vi "GenerateUUID.vi"(8 "error in (no error)":errorcluster) -> (0 "error out":errorcluster, 2 "UUID":string)   [LabVIEW 2019, in "Memory Data Access.lvlib"]
uses:
  Memory Data Access.lvlib
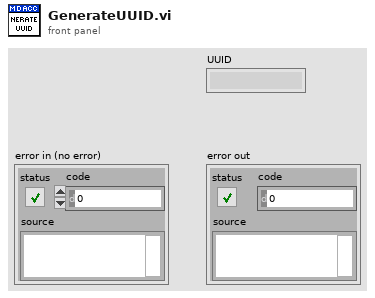
[diagram p1: front panel]
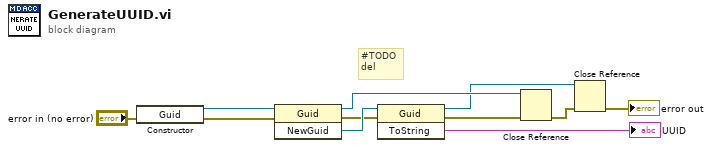
[diagram p0: block diagram]
diagram:
  # "#TODO\ndel"
  n1 = constructor class="Guid" ("Constructor Node")(error in="error in (no error)") -> (reference out=w11:refnum<k24>, error out=w10:errorcluster)  [unwired: 2 in, 1 out]
  n2 = invoke on="Invoke Node" class="Guid" method="NewGuid"(reference=w11, error in=w10) -> (reference out=w7:refnum<k24>, error out=w8:errorcluster, "NewGuid"=w9:refnum<k24>)  [unwired: 1 in]
  n3 = invoke on="Invoke Node" class="Guid" method="ToString"(reference=w9, error in=w8) -> (reference out=w4:refnum<k24>, error out=w6:errorcluster, "ToString"=→"UUID":string)  [unwired: 1 in]
  n4 = Close Reference(reference=w7, error in (no error)=w6) -> (error out=w5:errorcluster)
  n5 = Close Reference(reference=w4, error in (no error)=w5) -> (error out=→"error out":errorcluster)
